vi "Reports.Results CSV Data to Test Result V2 JSON.vi"(4 "File Data Objs":T1[](array[typedef]), 5 "CSV File":path) -> (1 "Test Result V2":T2={"Type"="TestExec Results", "Version"="2.0.0", "TestEvent"={"ProcessStep"="", "StartTime"="", "EndTime"="", "Mode"="Production", "Operator"="", "Comment"="", "Result"={"State"="", "Code"=0, "Desc"="", "Details"=""}}, "UUTInfo"={"Product"="", "Description"="", "PN"="", "SN"="", "LotNumber"="", "DateCode"="", "AltID"="", "Revision"="", "Properties"=[]}, "Station"={"Name"="", "Location"="", "ConfigID"="", "PCName"="", "Slot"=""}, "TestSequence"={"Name"="", "Setup"=[]}, "ResultData"=[], "DataObjs"=[]})   [LabVIEW 2018]
uses:
  Report.Result Data JSON V2.0.0.ctl
  Report.Result Test Event.ctl
  Report.Result State.ctl
  Report.Result UUTInfo.ctl
  Report.Result Test Station.ctl
  Report.Result Test Sequence.ctl
  Report.Result Measurement JSON Safe.ctl
  Report.Result DataObject.ctl
  Report.Result FileDataObject.ctl
  Time/Time.Format Selector.ctl
  <vilib>/KATE/Files/File Utils.lvlib
panel:
  out "Header":string[](array[string])
  out "Data":string[][](array[string])
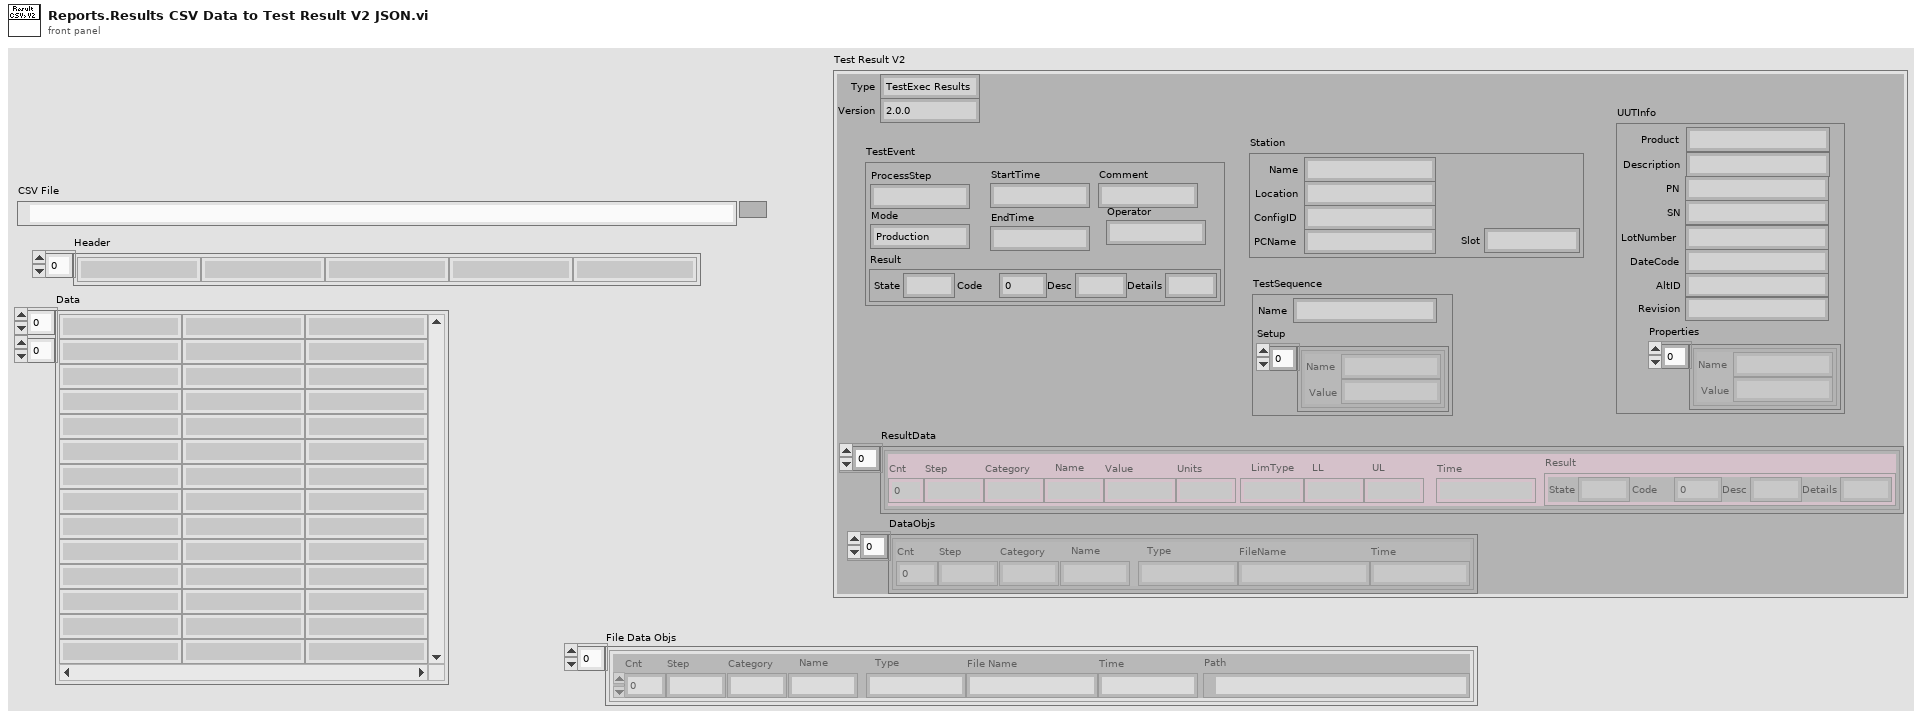
[diagram p1: front panel]
types:
  T1 = typedef "Report.Result FileDataObject.ctl" = cluster{"Cnt":i32, "Step":string, "Category":string, "Name":string, "Type":string, "File Name":string, "Time":string, "Path":path}
  T2 = typedef "Report.Result Data JSON V2.0.0.ctl" = cluster{"Type":string, "Version":string, "TestEvent":T3, "UUTInfo":T5, "Station":T6, "TestSequence":T7, "ResultData":T8[], "DataObjs":T9[]}
  T3 = typedef "Report.Result Test Event.ctl" = cluster{"ProcessStep":string, "StartTime":string, "EndTime":string, "Mode":string, "Operator":string, "Comment":string, "Result":T4}
  T4 = typedef "Report.Result State.ctl" = cluster{"State":string, "Code":i32, "Desc":string, "Details":string}
  T5 = typedef "Report.Result UUTInfo.ctl" = cluster{"Product":string, "Description":string, "PN":string, "SN":string, "LotNumber":string, "DateCode":string, "AltID":string, "Revision":string, "Properties":cluster{"Name":string, "Value":string}[]}
  T6 = typedef "Report.Result Test Station.ctl" = cluster{"Name":string, "Location":string, "ConfigID":string, "PCName":string, "Slot":string}
  T7 = typedef "Report.Result Test Sequence.ctl" = cluster{"Name":string, "Setup":cluster{"Name":string, "Value":string}[]}
  T8 = typedef "Report.Result Measurement JSON Safe.ctl" = cluster{"Cnt":i32, "Step":string, "Category":string, "Name":string, "Value":string, "Units":string, "LimType":string, "LL":string, "UL":string, "Time":string, "Result":T4}
  T9 = typedef "Report.Result DataObject.ctl" = cluster{"Cnt":i32, "Step":string, "Category":string, "Name":string, "Type":string, "FileName":string, "Time":string}
  T10 = typedef "Time.Format Selector.ctl" = enum16{"yyyy/mm/dd HH:MM:S.sss", "yyyy-MM-ddTHH:mm:ss[.mmm]"}
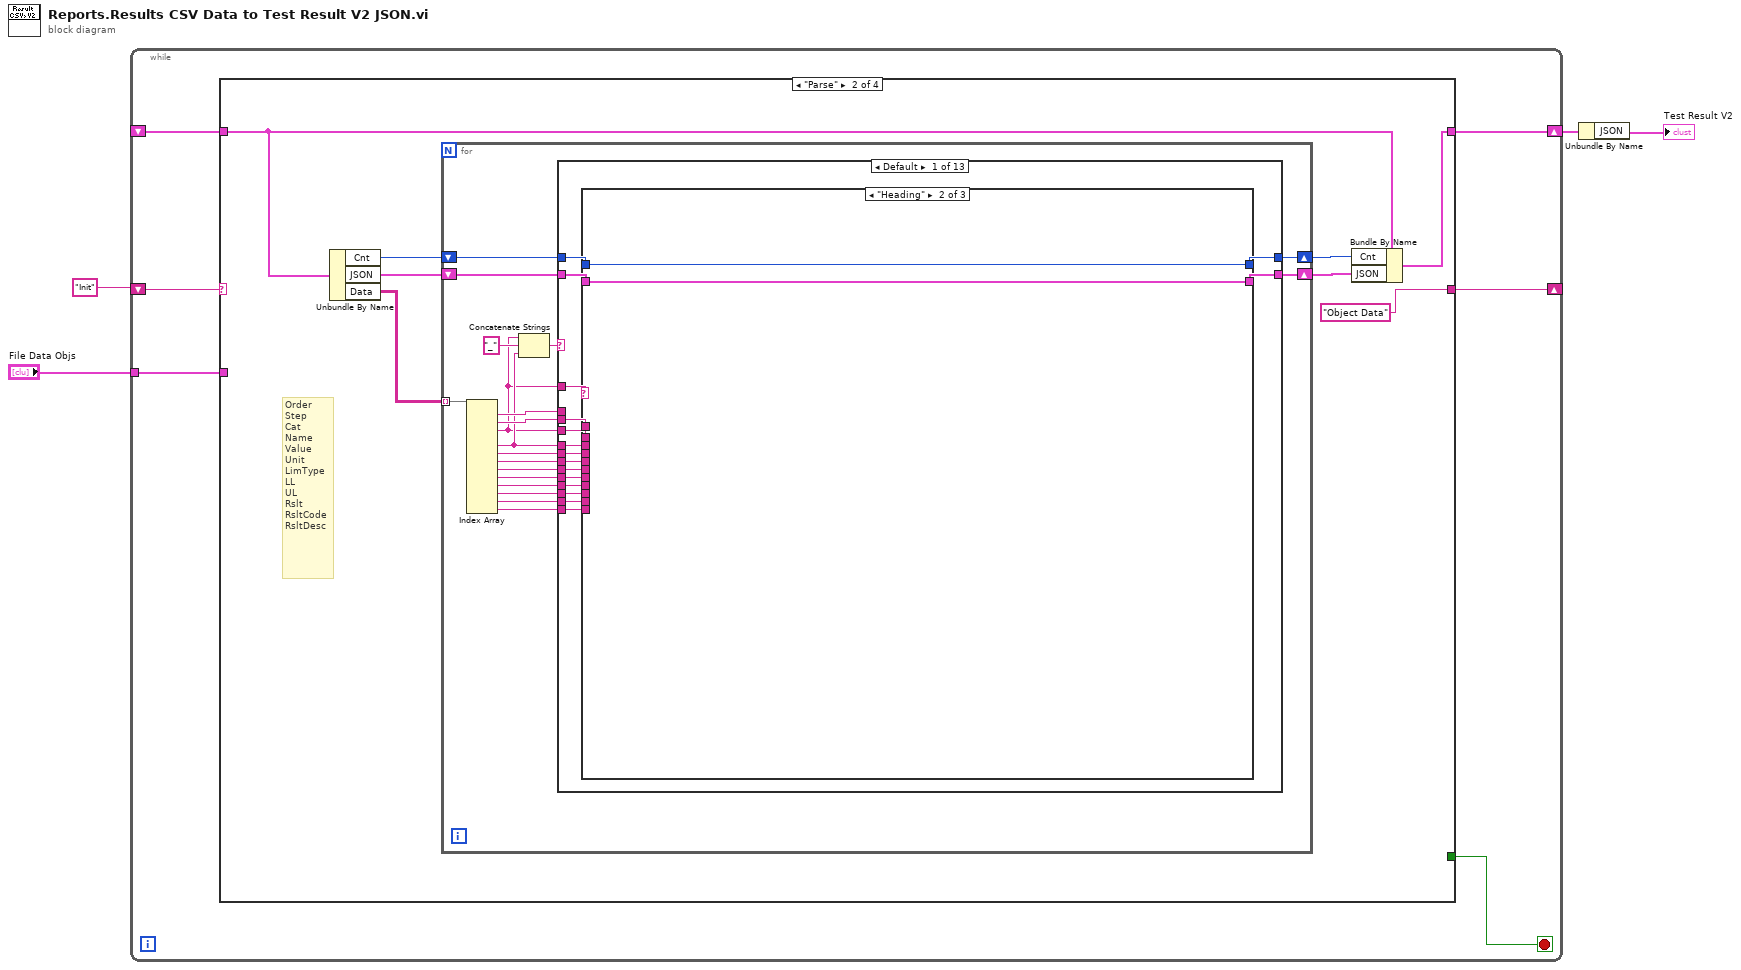
[diagram p0: block diagram]
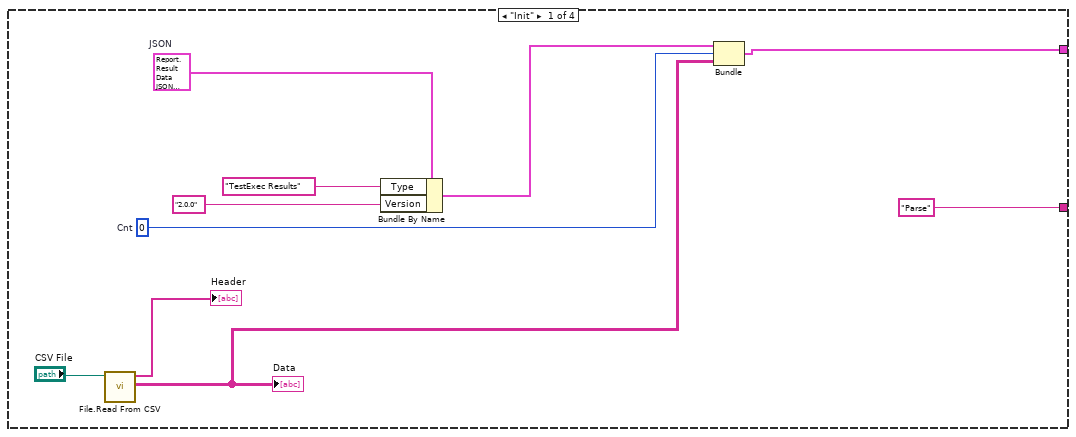
[diagram p2: hidden frame]
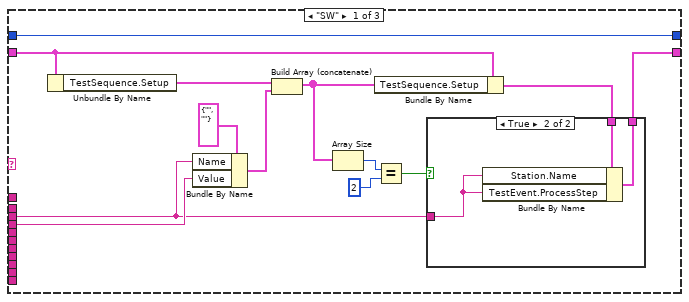
[diagram p3: hidden frame]
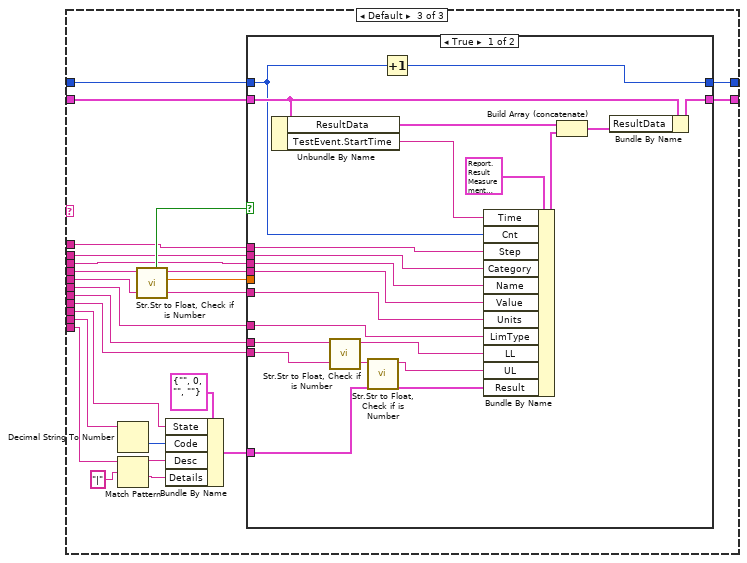
[diagram p5: hidden frame]
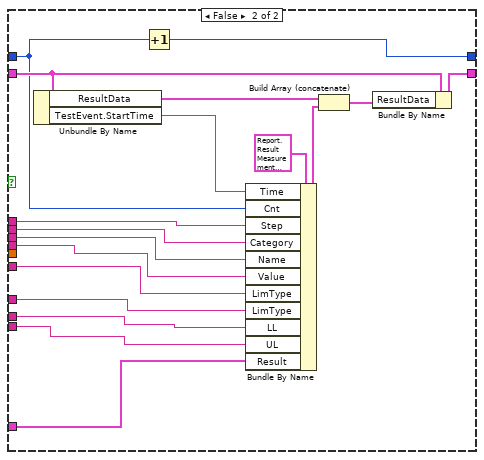
[diagram p6: hidden frame]
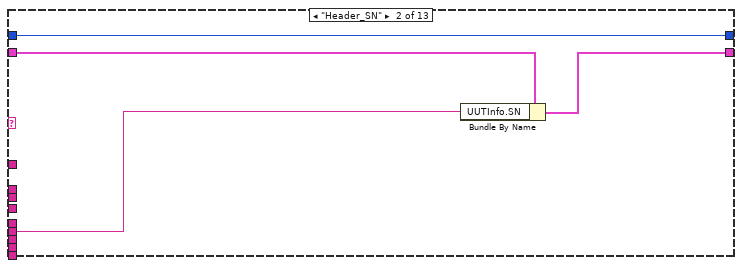
[diagram p7: hidden frame]
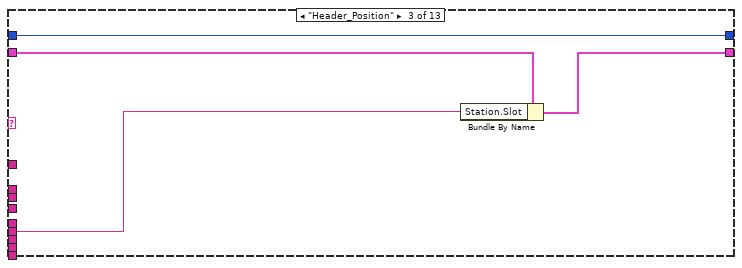
[diagram p8: hidden frame]
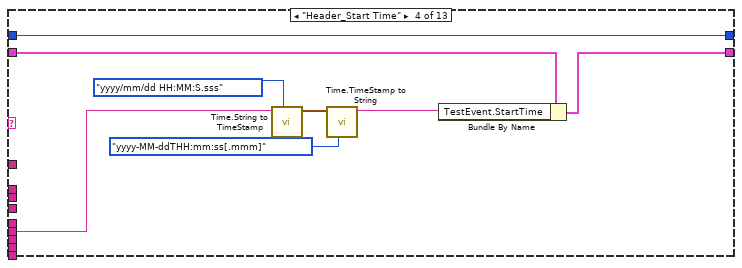
[diagram p9: hidden frame]
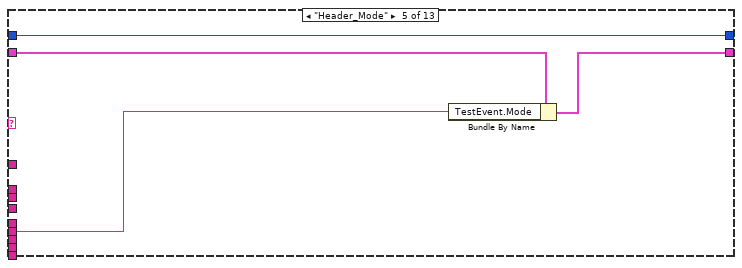
[diagram p10: hidden frame]
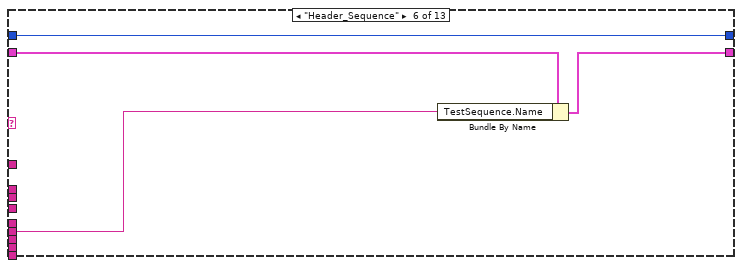
[diagram p11: hidden frame]
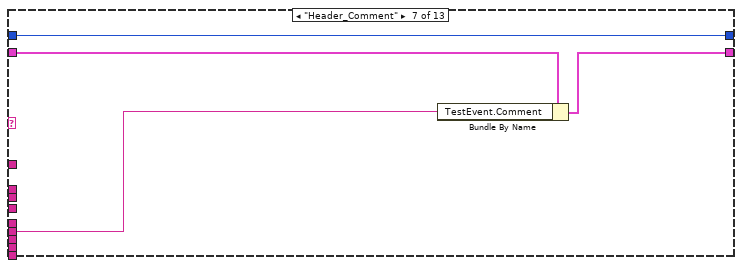
[diagram p12: hidden frame]
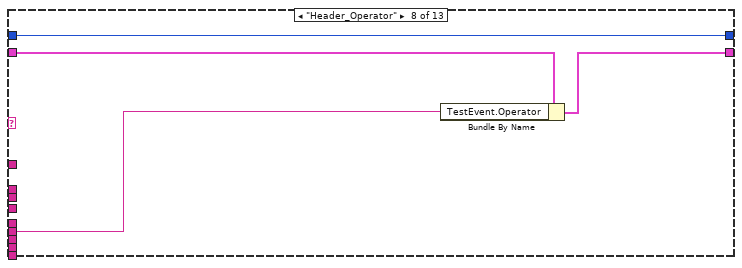
[diagram p13: hidden frame]
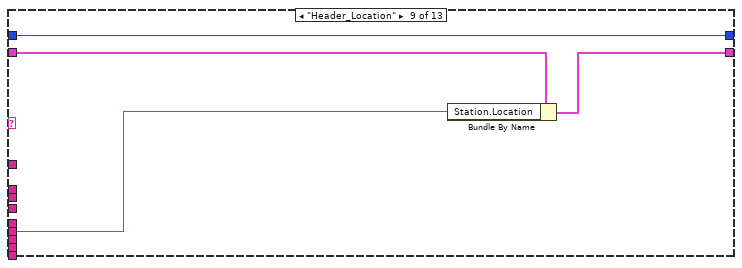
[diagram p14: hidden frame]
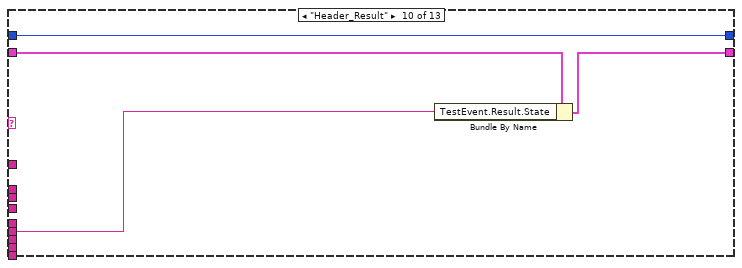
[diagram p15: hidden frame]
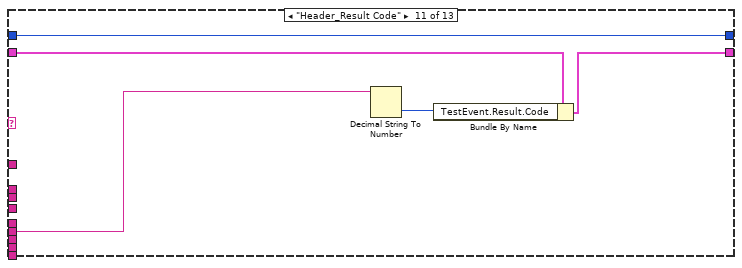
[diagram p16: hidden frame]
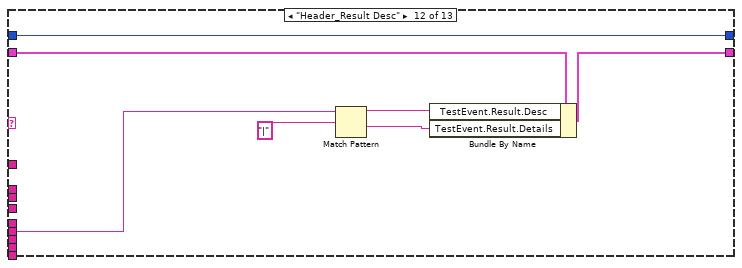
[diagram p17: hidden frame]
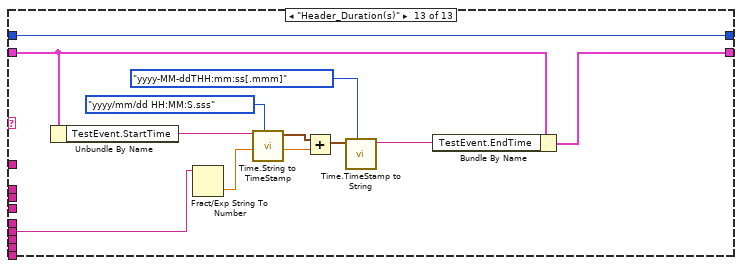
[diagram p18: hidden frame]
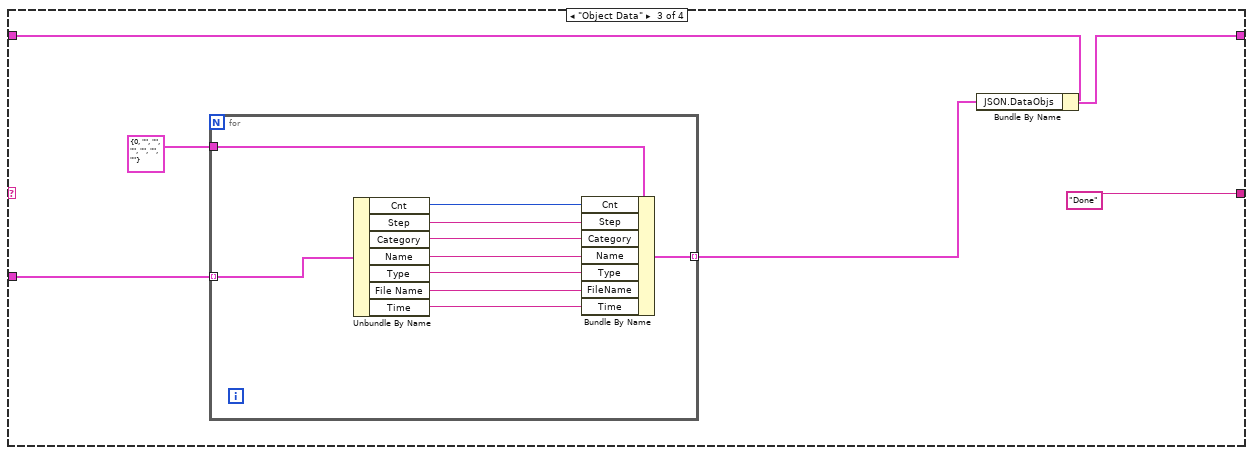
[diagram p19: hidden frame]
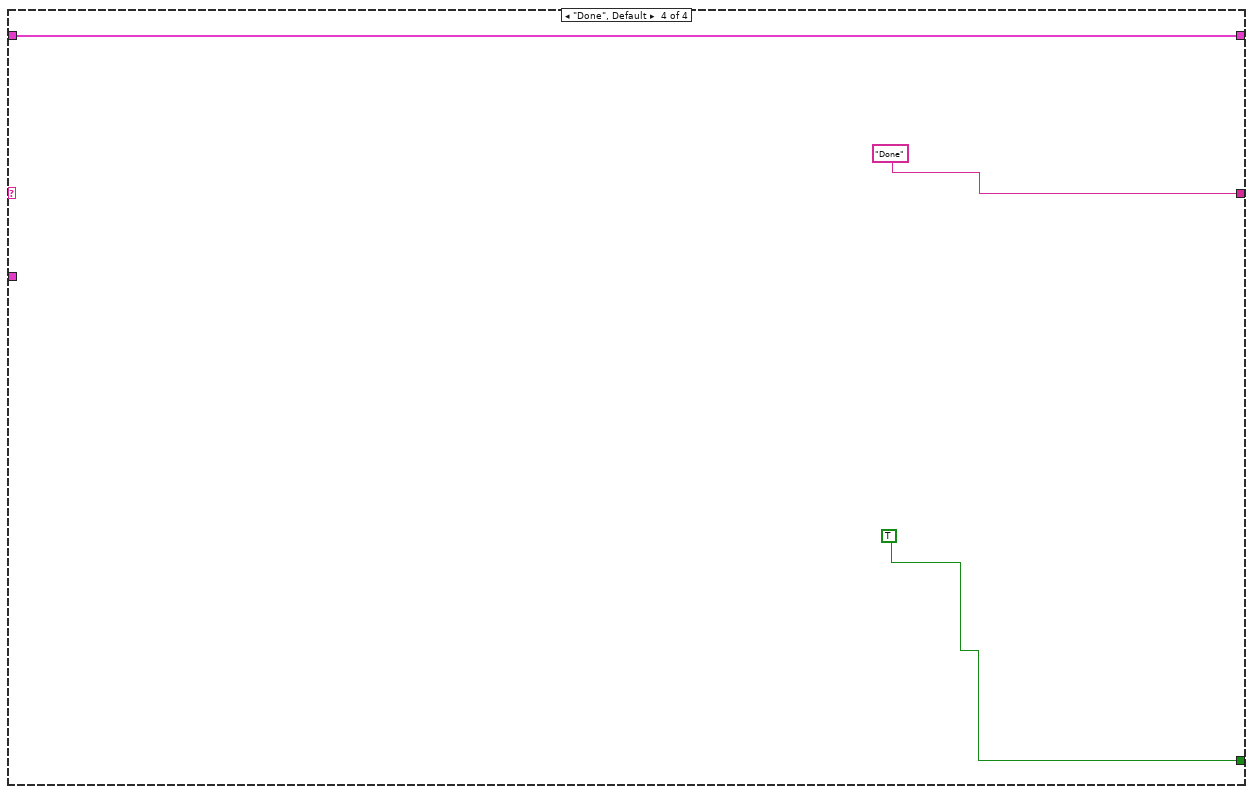
[diagram p20: hidden frame]
diagram:
  n1 = while {
    shift-right: [w5] -> w1
    shift-left: _ -> [w10]
    shift-right: [w7] -> _
    shift-left: "Init" -> [w8]
    tunnel: "File Data Objs" -> [w6]
    stop <- w9 stop-if-true
    n2 = case shown="\"Parse\"" w8 {
      tunnel: w10 -> [_ w25 w208 w226]
      tunnel: [w12 w22 w213 w226] -> w5
      tunnel: [_ _ _ TRUE] -> w9
      tunnel: ["Parse" ("Version") "Object Data" ("Version") "Done" ("Version") "Done"] -> w7
      tunnel: w6 -> [_ _ w209 _]
      frame "Init" {
        w11 = T2 {"Type"="TestExec Results", "Version"="2.0.0", "TestEvent"={"ProcessStep"="", "StartTime"="", "EndTime"="", "Mode"="Production", "Operator"="", "Comment"="", "Result"={"State"="", "Code"=0, "Desc"="", "Details"=""}}, "UUTInfo"={"Product"="", "Description"="", "PN"="", "SN"="", "LotNumber"="", "DateCode"="", "AltID"="", "Revision"="", "Properties"=[]}, "Station"={"Name"="", "Location"="", "ConfigID"="", "PCName"="", "Slot"=""}, "TestSequence"={"Name"="", "Setup"=[]}, "ResultData"=[], "DataObjs"=[]}  # JSON
        w16 = 0  # Cnt
        n3 = call <vilib>:"File.Read From CSV.vi"("File"="CSV File") -> ("Data"=w13:string[][], "Header"=→"Header":string[])  [unwired: 8 in, 1 out]
        "Data" <- w13
        n4 = Bundle By Name(cluster=w11, "Type"="TestExec Results", "Version"="2.0.0") -> (w17:T2)
        n5 = Bundle("JSON"=w17, "Cnt"=w16, "Data"=w13) -> (w12:cluster{"JSON":T2, "Cnt":i32, "Data":string[][]})  [unwired: 1 in]
      }
      frame "Parse" {
        # "Order\nStep\nCat\nName\nValue\nUnit\nLimType\nLL\nUL\nRslt\nRsltCode\nRsltDesc"
        n6 = Unbundle By Name(w25) -> ("Cnt"=w26:i32, "JSON"=w28:T2, "Data"=w27:string[][])
        n7 = for {
          shift-right: [w32] -> w24
          shift-left: w28 -> [w33]
          tunnel: w27 -> [w47] mode=indexing
          shift-right: [w30] -> w23
          shift-left: w26 -> [w31]
          n8 = Index Array(array=w47) -> (element #1=w44:string, element #2=w43:string, element #3=w29:string, element #4=w42:string, element #5=w41:string, element #6=w40:string, element #7=w39:string, element #8=w38:string, element #9=w37:string, element #10=w36:string, element #11=w35:string, element #12=w34:string)  [unwired: 12 in]
          n9 = Concatenate Strings(w29, "_", w42) -> (w45:string)
          n10 = case shown="Default" w45 {
            tunnel: w44 -> [_ _ _ _ _ _ _ _ _ _ _ _ _]
            tunnel: w43 -> [w58 _ _ _ _ _ _ _ _ _ _ _ _]
            tunnel: w29 -> [w57 _ _ _ _ _ _ _ _ _ _ _ _]
            tunnel: w42 -> [w56 _ _ _ _ _ _ _ _ _ _ _ _]
            tunnel: w41 -> [w61 w146 w150 w157 w162 w166 w170 w174 w178 w182 w186 w190 w204]
            tunnel: w40 -> [w55 _ _ _ _ _ _ _ _ _ _ _ _]
            tunnel: w39 -> [w54 _ _ _ _ _ _ _ _ _ _ _ _]
            tunnel: w38 -> [w53 _ _ _ _ _ _ _ _ _ _ _ _]
            tunnel: w37 -> [w52 _ _ _ _ _ _ _ _ _ _ _ _]
            tunnel: w36 -> [w49 _ _ _ _ _ _ _ _ _ _ _ _]
            tunnel: w35 -> [w51 _ _ _ _ _ _ _ _ _ _ _ _]
            tunnel: w34 -> [w50 _ _ _ _ _ _ _ _ _ _ _ _]
            tunnel: w33 -> [w63 w148 w152 w160 w164 w168 w172 w176 w180 w184 w189 w196 w205]
            tunnel: [w62 w147 w151 w159 w163 w167 w171 w175 w179 w183 w188 w195 w207] -> w32
            tunnel: w31 -> [w60 w145 w149 w158 w161 w165 w169 w173 w177 w181 w187 w194 w206]
            tunnel: [w59 w145 w149 w158 w161 w165 w169 w173 w177 w181 w187 w194 w206] -> w30
            tunnel: w29 -> [w48 _ _ _ _ _ _ _ _ _ _ _ _]
            frame Default {
              n11 = case shown="\"Heading\"" w48 {
                tunnel: w63 -> [w75 w81 w106]
                tunnel: [w65 w81 w105] -> w62
                tunnel: w61 -> [w72 _ w104]
                tunnel: w60 -> [w76 w82 w103]
                tunnel: [w76 w82 w102] -> w59
                tunnel: w58 -> [_ _ w100]
                tunnel: w57 -> [_ _ w99]
                tunnel: w56 -> [w64 _ w98]
                tunnel: w55 -> [_ _ w95]
                tunnel: w54 -> [_ _ w94]
                tunnel: w53 -> [_ _ w93]
                tunnel: w52 -> [_ _ w92]
                tunnel: w51 -> [_ _ w91]
                tunnel: w50 -> [_ _ w86]
                tunnel: w49 -> [_ _ w84]
                frame "SW" {
                  n12 = Unbundle By Name(w75) -> ("TestSequence.Setup"=w71:cluster{"Name":string, "Value":string}[])
                  n13 = Bundle By Name(cluster=cluster{"Name":string, "Value":string} {"Name"="", "Value"=""} ("Setup"), "Name"=w64, "Value"=w72) -> (w73:cluster{"Name":string, "Value":string})
                  n14 = Build Array (concatenate)(w71, w73) -> (w68:cluster{"Name":string, "Value":string}[])
                  n15 = Array Size(array=w68) -> (size(s)=w70:i32)
                  n16 = Bundle By Name(cluster=w75, "TestSequence.Setup"=w68) -> (w66:T2)
                  n17 = Equal?(x=w70, y=2) -> (x = y?=w67:bool)
                  n18 = case shown="True" w67 {
                    tunnel: w66 -> [w77 w80]
                    tunnel: [w77 w79] -> w65
                    tunnel: w64 -> [_ w78]
                    frame False {
                    }
                    frame True {
                      n19 = Bundle By Name(cluster=w80, "Station.Name"=w78, "TestEvent.ProcessStep"=w78) -> (w79:T2)
                    }
                  }
                }
                frame "Heading" {
                }
                frame Default {
                  n20 = Decimal String To Number(string=w91) -> (number=w85:i32)  [unwired: 2 in, 1 out]
                  n21 = Match Pattern(string=w86, regular expression="|") -> (before substring=w89:string, after substring=w90:string)  [unwired: 1 in, 2 out]
                  n22 = call "Str.Str to Float, Check if is Number.vi"("Value In"=w104) -> ("Num Out"=w96:dbl, "Value Out"=w97:string, "Is Num"=w101:bool)  [unwired: 8 in]
                  n23 = Bundle By Name(cluster=T4 {"State"="", "Code"=0, "Desc"="", "Details"=""} ("Result"), "State"=w84, "Code"=w85, "Desc"=w89, "Details"=w90) -> (w83:T4)
                  n24 = case shown="True" w101 {
                    tunnel: w106 -> [w124 w142]
                    tunnel: [w126 w144] -> w105
                    tunnel: w103 -> [w120 w138]
                    tunnel: [w125 w143] -> w102
                    tunnel: w100 -> [w119 w137]
                    tunnel: w99 -> [w118 w136]
                    tunnel: w98 -> [w117 w135]
                    tunnel: w97 -> [w109 w130]
                    tunnel: w96 -> [_ _]
                    tunnel: w95 -> [w116 w134]
                    tunnel: w94 -> [w111 w131]
                    tunnel: w93 -> [w113 w129]
                    tunnel: w92 -> [w114 w128]
                    tunnel: w83 -> [w115 w133]
                    frame True {
                      n25 = Unbundle By Name(w124) -> ("ResultData"=w123:T8[], "TestEvent.StartTime"=w112:string)
                      n26 = call "Str.Str to Float, Check if is Number.vi"("Value In"=w113) -> ("Value Out"=w108:string)  [unwired: 8 in, 2 out]
                      n27 = call "Str.Str to Float, Check if is Number.vi"("Value In"=w114) -> ("Value Out"=w107:string)  [unwired: 8 in, 2 out]
                      n28 = Increment(x=w120) -> (x+1=w125:i32)
                      n29 = Bundle By Name(cluster=T8 {"Cnt"=0, "Step"="", "Category"="", "Name"="", "Value"="", "Units"="", "LimType"="", "LL"="", "UL"="", "Time"="", "Result"={"State"="", "Code"=0, "Desc"="", "Details"=""}} ("Measurement 2"), "Time"=w112, "Cnt"=w120, "Step"=w119, "Category"=w118, "Name"=w117, "Value"=w109, "Units"=w116, "LimType"=w111, "LL"=w108, "UL"=w107, "Result"=w115) -> (w121:T8)
                      n30 = Build Array (concatenate)(w123, w121) -> (w122:T8[])
                      n31 = Bundle By Name(cluster=w124, "ResultData"=w122) -> (w126:T2)
                    }
                    frame False {
                      n32 = Unbundle By Name(w142) -> ("ResultData"=w141:T8[], "TestEvent.StartTime"=w132:string)
                      n33 = Increment(x=w138) -> (x+1=w143:i32)
                      n34 = Bundle By Name(cluster=T8 {"Cnt"=0, "Step"="", "Category"="", "Name"="", "Value"="", "Units"="", "LimType"="", "LL"="", "UL"="", "Time"="", "Result"={"State"="", "Code"=0, "Desc"="", "Details"=""}} ("Measurement 2"), "Time"=w132, "Cnt"=w138, "Step"=w137, "Category"=w136, "Name"=w135, "Value"=w130, "LimType"=w134, "LimType"=w131, "LL"=w129, "UL"=w128, "Result"=w133) -> (w139:T8)
                      n35 = Build Array (concatenate)(w141, w139) -> (w140:T8[])
                      n36 = Bundle By Name(cluster=w142, "ResultData"=w140) -> (w144:T2)
                    }
                  }
                }
              }
            }
            frame "Header_SN" {
              n37 = Bundle By Name(cluster=w148, "UUTInfo.SN"=w146) -> (w147:T2)
            }
            frame "Header_Position" {
              n38 = Bundle By Name(cluster=w152, "Station.Slot"=w150) -> (w151:T2)
            }
            frame "Header_Start Time" {
              n39 = call "Time.String to TimeStamp.vi"("TimeFormat"=Time.Format_Selector."yyyy/mm/dd HH:MM:S.sss", "Time String In"=w157) -> ("Time Stamp Out"=w156:timestamp)  [unwired: 9 in]
              n40 = call "Time.TimeStamp to String.vi"("TimeFormat"=Time.Format_Selector."yyyy-MM-ddTHH:mm:ss[.mmm]", "Time Stamp in"=w156) -> ("Time String Out"=w155:string)  [unwired: 9 in]
              n41 = Bundle By Name(cluster=w160, "TestEvent.StartTime"=w155) -> (w159:T2)
            }
            frame "Header_Mode" {
              n42 = Bundle By Name(cluster=w164, "TestEvent.Mode"=w162) -> (w163:T2)
            }
            frame "Header_Sequence" {
              n43 = Bundle By Name(cluster=w168, "TestSequence.Name"=w166) -> (w167:T2)
            }
            frame "Header_Comment" {
              n44 = Bundle By Name(cluster=w172, "TestEvent.Comment"=w170) -> (w171:T2)
            }
            frame "Header_Operator" {
              n45 = Bundle By Name(cluster=w176, "TestEvent.Operator"=w174) -> (w175:T2)
            }
            frame "Header_Location" {
              n46 = Bundle By Name(cluster=w180, "Station.Location"=w178) -> (w179:T2)
            }
            frame "Header_Result" {
              n47 = Bundle By Name(cluster=w184, "TestEvent.Result.State"=w182) -> (w183:T2)
            }
            frame "Header_Result Code" {
              n48 = Decimal String To Number(string=w186) -> (number=w185:i32)  [unwired: 2 in, 1 out]
              n49 = Bundle By Name(cluster=w189, "TestEvent.Result.Code"=w185) -> (w188:T2)
            }
            frame "Header_Result Desc" {
              n50 = Match Pattern(string=w190, regular expression="|") -> (before substring=w192:string, after substring=w191:string)  [unwired: 1 in, 2 out]
              n51 = Bundle By Name(cluster=w196, "TestEvent.Result.Desc"=w192, "TestEvent.Result.Details"=w191) -> (w195:T2)
            }
            frame "Header_Duration(s)" {
              n52 = Unbundle By Name(w205) -> ("TestEvent.StartTime"=w203:string)
              n53 = Fract/Exp String To Number(string=w204) -> (number=w201:dbl)  [unwired: 3 in, 1 out]
              n54 = call "Time.String to TimeStamp.vi"("TimeFormat"=Time.Format_Selector."yyyy/mm/dd HH:MM:S.sss", "Time String In"=w203) -> ("Time Stamp Out"=w202:timestamp)  [unwired: 9 in]
              n55 = Add(x=w202, y=w201) -> (x+y=w200:timestamp)
              n56 = call "Time.TimeStamp to String.vi"("TimeFormat"=Time.Format_Selector."yyyy-MM-ddTHH:mm:ss[.mmm]", "Time Stamp in"=w200) -> ("Time String Out"=w199:string)  [unwired: 9 in]
              n57 = Bundle By Name(cluster=w205, "TestEvent.EndTime"=w199) -> (w207:T2)
            }
          }
        }
        n58 = Bundle By Name(cluster=w25, "Cnt"=w23, "JSON"=w24) -> (w22:cluster{"JSON":T2, "Cnt":i32, "Data":string[][]})
      }
      frame "Object Data" {
        n59 = for {
          tunnel: w209 -> [w221] mode=indexing
          tunnel: T9 {"Cnt"=0, "Step"="", "Category"="", "Name"="", "Type"="", "FileName"="", "Time"=""} ("Data Object") -> [w223]
          tunnel: [w222] -> w211 mode=indexing
          n60 = Unbundle By Name(w221) -> ("Cnt"=w220:i32, "Step"=w219:string, "Category"=w218:string, "Name"=w217:string, "Type"=w216:string, "File Name"=w215:string, "Time"=w214:string)
          n61 = Bundle By Name(cluster=w223, "Cnt"=w220, "Step"=w219, "Category"=w218, "Name"=w217, "Type"=w216, "FileName"=w215, "Time"=w214) -> (w222:T9)
        }
        n62 = Bundle By Name(cluster=w208, "JSON.DataObjs"=w211) -> (w213:cluster{"JSON":T2, "Cnt":i32, "Data":string[][]})
      }
      frame "Done", Default {
      }
    }
  }
  n63 = Unbundle By Name(w1) -> ("JSON"=→"Test Result V2":T2)
